vi "Calcu_Torque Weight.vi"(6 "Resolution":string[][](array[string]), 8 "Weight Set":string[][][](array[string]), 9 "torque arm":dbl, 10 "STD Data":string[][](array[string]), 11 "Condition":string[][](array[string])) -> (0 "기타정보":string[][](array[string]), 1 "Condition Out":string[][](array[string]), 2 "분동조합":string[][](array[string]), 3 "분동질량(kg)":string[][](array[string]))   [LabVIEW 2020]
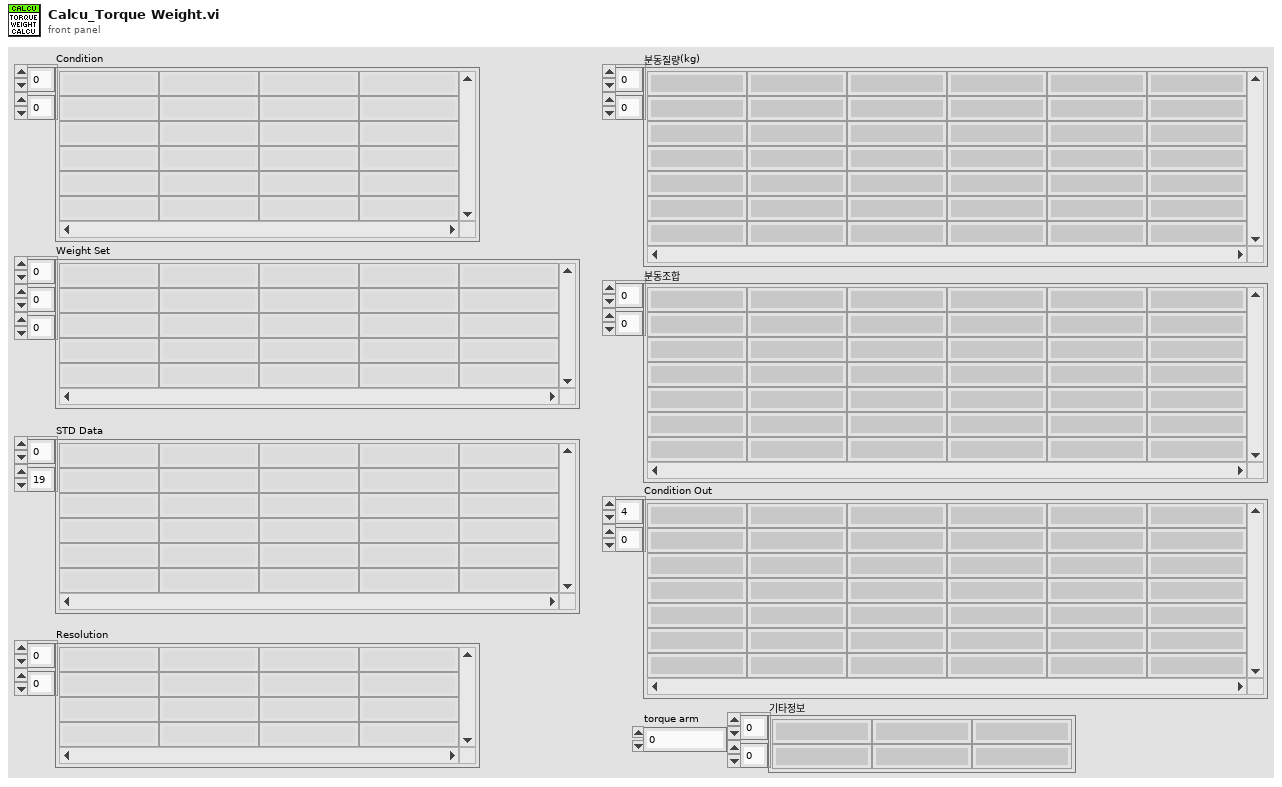
[diagram p1: front panel]
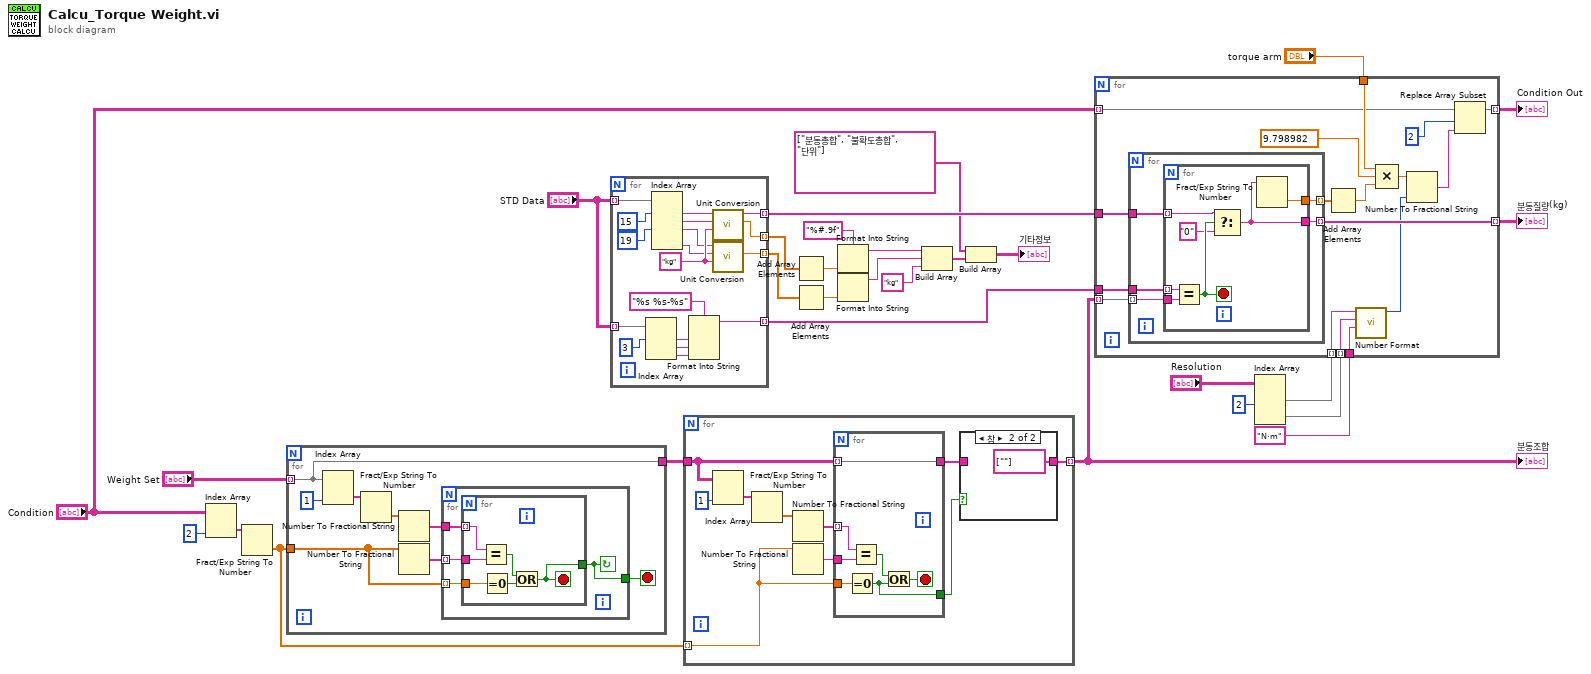
[diagram p0: block diagram]
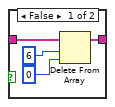
[diagram p2: hidden frame]
diagram:
  w4 = "%#.9f" ("포맷 문자열")
  n1 = Index Array(array="Condition", index (col)=2 ("비활성화된 인덱스 (열)")) -> (element=w27:string[])  [unwired: 1 in]
  n2 = Fract/Exp String To Number(string=w27) -> (number=w26:dbl[])  [unwired: 3 in, 1 out]
  n3 = for {
    tunnel: "Weight Set" -> [w31] mode=indexing
    tunnel: w26 -> [w30]
    tunnel: [w31] -> w25
    stop <- w33 stop-if-true
    n4 = Index Array(array=w31, index (col)=1 ("비활성화된 인덱스 (열)")) -> (element=w36:string[])  [unwired: 1 in]
    n5 = Fract/Exp String To Number(string=w36) -> (number=w35:dbl[])  [unwired: 3 in, 1 out]
    n6 = Number To Fractional String(number=w35) -> (F-format string=w32:string[])  [unwired: 3 in]
    n7 = Number To Fractional String(number=w30) -> (F-format string=w34:string[])  [unwired: 3 in]
    n8 = for {
      tunnel: w34 -> [w41] mode=indexing
      tunnel: w32 -> [w40]
      tunnel: [w38] -> w33
      tunnel: w30 -> [w39] mode=indexing
      stop <- w38 continue-if-true
      n9 = for {
        tunnel: w41 -> [w47]
        tunnel: w40 -> [w46] mode=indexing
        tunnel: w39 -> [w45]
        tunnel: [w42] -> w38
        stop <- w42 stop-if-true
        n10 = Equal?(x=w46, y=w47) -> (x = y?=w43:bool)
        n11 = Equal To 0?(x=w45) -> (x = 0?=w44:bool)
        n12 = Or(x=w43, y=w44) -> (x .or. y?=w42:bool)
      }
    }
  }
  n13 = for {
    tunnel: "STD Data" -> [w65] mode=indexing
    tunnel: [w59] -> w23 mode=indexing
    tunnel: "STD Data" -> [w58] mode=indexing
    tunnel: [w51] -> w21 mode=indexing
    tunnel: [w50] -> w11 mode=indexing
    tunnel: [w49] -> w10 mode=indexing
    w53 = "kg" ("환산단위")
    n14 = Index Array(array=w65, index #1=3 ("인덱스")) -> (element #1=w63:string, element #2=w62:string, element #3=w61:string)  [unwired: 2 in]
    n15 = Index Array(array=w58, index #1=15 ("인덱스"), index #3=19 ("인덱스")) -> (element #1=w56:string, element #2=w55:string, element #3=w52:string, element #5=w48:string)  [unwired: 3 in, 1 out]
    n16 = Format Into String(format string="%s %s-%s" ("포맷 문자열"), w63, w62, w61) -> (resulting string=w59:string)  [unwired: 2 in, 1 out]
    n17 = call "Unit Conversion.vi"("환산단위"=w53, "입력단위"=w55, "입력값"=w56) -> ("환산값 (DBL)"=w50:dbl, "환산값 (string)"=w51:string)  [unwired: 3 in, 4 out]
    n18 = call "Unit Conversion.vi"("환산단위"=w53, "입력단위"=w48, "입력값"=w52) -> ("환산값 (DBL)"=w49:dbl)  [unwired: 3 in, 5 out]
  }
  n19 = for {
    tunnel: w25 -> [w69]
    tunnel: w26 -> [w71] mode=indexing
    tunnel: [w67] -> w24 mode=indexing
    n20 = Index Array(array=w69, index (col)=1 ("비활성화된 인덱스 (열)")) -> (element=w75:string[])  [unwired: 1 in]
    n21 = Fract/Exp String To Number(string=w75) -> (number=w74:dbl[])  [unwired: 3 in, 1 out]
    n22 = Number To Fractional String(number=w74) -> (F-format string=w72:string[])  [unwired: 3 in]
    n23 = Number To Fractional String(number=w71) -> (F-format string=w73:string)  [unwired: 3 in]
    n24 = for {
      tunnel: w73 -> [w87]
      tunnel: w72 -> [w86] mode=indexing
      tunnel: w71 -> [w85]
      tunnel: w69 -> [w82] mode=indexing
      tunnel: [w82] -> w68
      tunnel: [w81] -> w66
      stop <- w83 stop-if-true
      n25 = Equal To 0?(x=w85) -> (x = 0?=w81:bool)
      n26 = Equal?(x=w86, y=w87) -> (x = y?=w84:bool)
      n27 = Or(x=w84, y=w81) -> (x .or. y?=w83:bool)
    }
    n28 = case shown="참" w66 {
      tunnel: w68 -> [w79 _]
      tunnel: [w78 string[] [""] ("Weight Set")] -> w67
      frame False {
        n29 = Delete From Array(array=w79, length=6 ("인덱스"), index=0 ("인덱스")) -> (array with subset deleted=w78:string[])  [unwired: 1 out]
      }
      frame True {
      }
    }
  }
  "분동조합" <- w24
  n30 = Add Array Elements(numeric array=w11) -> (sum=w8:dbl)
  n31 = Add Array Elements(numeric array=w10) -> (sum=w5:dbl)
  n32 = Format Into String(format string=w4, w8) -> (resulting string=w7:string)  [unwired: 2 in, 1 out]
  n33 = Format Into String(format string=w4, w5) -> (resulting string=w6:string)  [unwired: 2 in, 1 out]
  n34 = Build Array(w7, w6, "kg" ("원소")) -> (w9:string[])
  n35 = Build Array(string[] ["분동총합", "불확도총합", "단위"] ("기타정보 2"), w9) -> (→"기타정보":string[][])
  n36 = Index Array(array="Resolution", index (col) #1=2 ("비활성화된 인덱스 (열)")) -> (element #1=w14:string[], element #2=w13:string[])  [unwired: 3 in]
  n37 = for {
    tunnel: w24 -> [w104] mode=indexing
    tunnel: w21 -> [w103]
    tunnel: w23 -> [w102]
    tunnel: [w101] -> w22 mode=indexing
    tunnel: "torque arm" -> [w96]
    tunnel: "Condition" -> [w94] mode=indexing
    tunnel: [w95] -> w17 mode=indexing
    tunnel: w14 -> [w93] mode=indexing
    tunnel: w13 -> [w92] mode=indexing
    tunnel: "N·m" ("기준단위") -> [w90]
    n38 = for {
      tunnel: w104 -> [w108] mode=indexing
      tunnel: w103 -> [w107]
      tunnel: w102 -> [w109]
      tunnel: [w106] -> w101 mode=indexing
      tunnel: [w105] -> w100 mode=indexing
      n39 = for {
        tunnel: w109 -> [w116] mode=indexing
        tunnel: w108 -> [w115]
        tunnel: w107 -> [w113] mode=indexing
        tunnel: [w111] -> w106
        tunnel: [w110] -> w105
        stop <- w114 stop-if-true
        n40 = Equal?(x=w116, y=w115) -> (x = y?=w114:bool)
        n41 = Select(t=w113, s=w114, f="0") -> (s? t:f=w111:string)
        n42 = Fract/Exp String To Number(string=w111) -> (number=w110:dbl)  [unwired: 3 in, 1 out]
      }
    }
    n43 = Add Array Elements(numeric array=w100) -> (sum=w99:dbl)
    n44 = call "Number Format.vi"("기준단위"=w90, "입력단위"=w92, "입력값"=w93) -> ("정밀도(단위적용)"=w88:i32)  [unwired: 8 in]
    n45 = Compound Arithmetic op=MULTIPLY(w96, 9.798982 ("y"), w99) -> (w91:dbl)
    n46 = Number To Fractional String(number=w91, precision (6)=w88) -> (F-format string=w89:string)  [unwired: 2 in]
    n47 = Replace Array Subset(array=w94, new element=w89, index=2 ("비활성화된 인덱스 (열)")) -> (w95:string[])
  }
  "분동질량(kg)" <- w22
  "Condition Out" <- w17
